vi "LinxI2cRead.vi"(5 "EOF":u8, 6 "Timeout (1000 ms)":u16=1000, 7 "I2C Channel":u8, 8 "Error In":errorcluster, 9 "Num Bytes":u8, 10 "Slave Address":u8, 11 "LINX Resource":T1) -> (0 "Error Out":errorcluster, 2 "Data":u8[](array[numeric]), 3 "LINX Resource":T1)   [LabVIEW 2019, in "LMH-LINX.lvlib" / "Local IO.lvlib"]
uses:
  <vilib>/MakerHub/LINX/Private/Local IO/Local IO.lvlib
  <vilib>/MakerHub/LINX/Private/Type Defs/LINX Ref.ctl
  <vilib>/MakerHub/LINX/Private/Type Defs/Platform.ctl
  <vilib>/MakerHub/LINX/Private/Type Defs/Interface.ctl
  <vilib>/MakerHub/LINX/Private/Device/Type Defs/LINX Device Config.ctl
  <vilib>/MakerHub/LINX/Private/Device/Type Defs/TCP Config.ctl
  <vilib>/MakerHub/LINX/Private/Device/Type Defs/Channels.ctl
  <vilib>/MakerHub/LINX/LMH-LINX.lvlib
  <vilib>/MakerHub/LINX/Private/Type Defs/Channel FGV States.ctl
  <vilib>/myRIO/Instrument Drivers/Onboard IO/I2C/typedefs/I2C Transfer Rate.ctl
  <vilib>/myRIO/Instrument Drivers/Onboard IO/I2C/typedefs/I2C Configuration.ctl
  <vilib>/myRIO/Common/Instrument Driver Framework/myRIO v1.0/I2C/typedefs/I2C Channels Enum.ctl
  <vilib>/myRIO/Common/Instrument Driver Framework/Utilities/typedefs/Generic FPGA Reference.ctl
  <vilib>/myRIO/Common/Instrument Driver Framework/Utilities/typedefs/myRIO v1.0 Reference.ctl
  <vilib>/myRIO/Common/Instrument Driver Framework/Utilities/typedefs/Hardware Version Enum.ctl
  <vilib>/myRIO/Common/Instrument Driver Framework/Utilities/typedefs/myRIO Generic Hardware Reference.ctl
  <vilib>/myRIO/Instrument Drivers/Onboard IO/I2C/typedefs/I2C Reference.ctl
  <vilib>/MakerHub/LINX/Resources/liblinxdevice.dll
  <vilib>/MakerHub/LINX/Private/Device/Device.lvlib
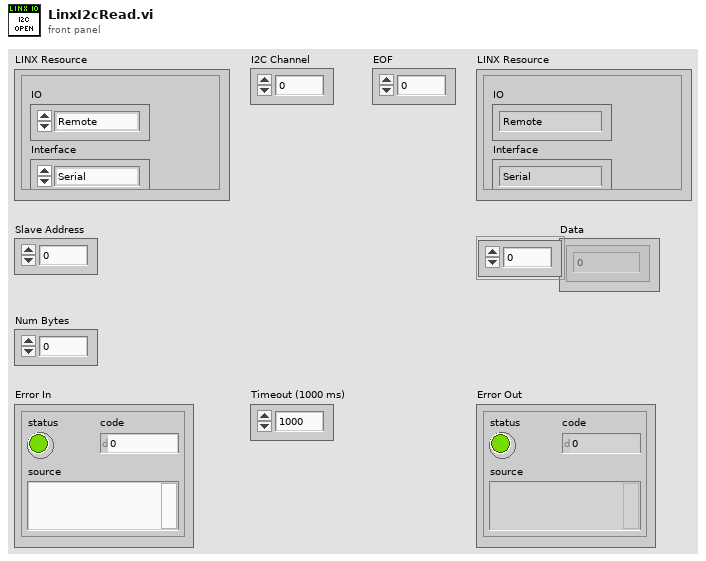
[diagram p1: front panel]
types:
  T1 = typedef "LMH-LINX.lvlib/LINX Ref.ctl" = cluster{"IO":T2, "Interface":T3, "LINX Device Config":T4}
  T2 = typedef "LMH-LINX.lvlib/Platform.ctl" = enum16{"Remote", "Local"}
  T3 = typedef "LMH-LINX.lvlib/Interface.ctl" = enum16{"Serial", "TCP"}
  T4 = typedef "LMH-LINX.lvlib/Device.lvlib/LINX Device Config.ctl" = cluster{"Interface":T3, "COM Port":refnum<visa-resource-name>, "TCP Configuration":T5, "Device Family":u8, "Device ID":u8, "Device Name":string, "TCP Ref":refnum<k5>, "Channels":T6}
  T5 = typedef "LMH-LINX.lvlib/Device.lvlib/TCP Config.ctl" = cluster{"IP Address":string, "Port":u16}
  T6 = typedef "LMH-LINX.lvlib/Channels.ctl" = cluster{"DI":u8[], "DO":u8[], "AI":u8[], "AO":u8[], "PWM":u8[], "QE":u8[], "UART":u8[], "I2C 2":u8[], "SPI":u8[], "CAN":u8[], "Servo":u8[], "AI Ref (V)":dbl, "AI Resolution (Bits)":u8, "AO Ref (V)":dbl, "AO Resolution (Bits)":u8}
  T7 = typedef "I2C.lvlib/I2C Reference.ctl" = cluster{"myRIO Reference":T8, "I2C Channels Enum":T12, "I2C Configuration":T13}
  T8 = typedef "myRIO Generic Hardware Reference.ctl" = cluster{"myRIO Model":T9, "myRIO Hardware Reference":T10}
  T9 = typedef "Hardware Version Enum.ctl" = enum16{"Unknown", "myRIO-1900", "myRIO-1950"}
  T10 = typedef "myRIO v1.0 Reference.ctl" = cluster{"Generic FPGA Reference":T11, "Allow multiple opens":bool}
  T11 = typedef "Generic FPGA Reference.ctl" = refnum<k20>
  T12 = typedef "I2C Channels Enum.ctl" = enum16{"Not Connected", "A/I2C", "B/I2C"}
  T13 = typedef "I2C.lvlib/I2C Configuration.ctl" = cluster{"I2C Transfer Rate":T14}
  T14 = typedef "I2C.lvlib/I2C Transfer Rate.ctl" = enum16{"Standard mode (100 kbps)", "Fast mode (400 kbps)"}
  T15 = typedef "LMH-LINX.lvlib/Channel FGV States.ctl" = enum16{"Initialize", "Get", "Set"}
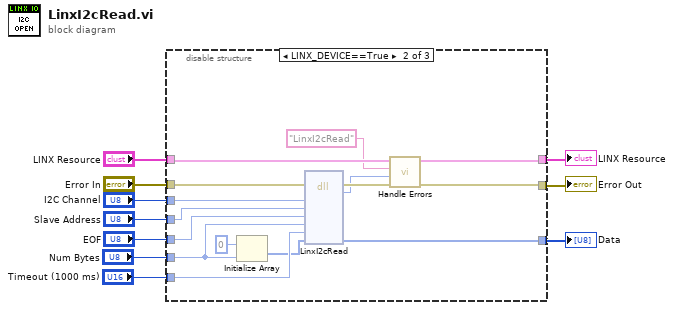
[diagram p0: block diagram]
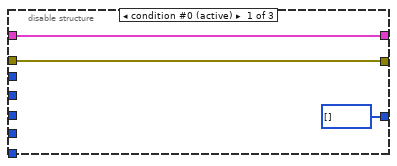
[diagram p2: hidden frame]
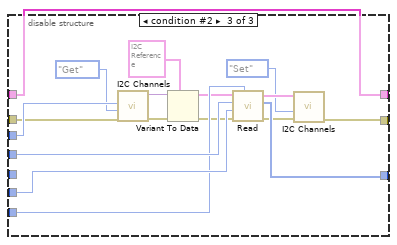
[diagram p3: hidden frame]
diagram:
  n1 = disable-structure shown="LINX_DEVICE==True" {
    disable-tunnel: "LINX Resource" -> [w13 w27 w44]
    disable-tunnel: "Error In" -> [w12 w28 w42]
    disable-tunnel: [w12 w25 w45] -> w8
    disable-tunnel: [w13 w26 w44] -> w7
    disable-tunnel: "I2C Channel" -> [_ w21 w43]
    disable-tunnel: "Slave Address" -> [_ w20 w41]
    disable-tunnel: "EOF" -> [_ w19 _]
    disable-tunnel: "Timeout (1000 ms)" -> [_ w18 w39]
    disable-tunnel: "Num Bytes" -> [_ w15 w40]
    disable-tunnel: [u8[] [] ("Data") w14 w38] -> w1
    frame condition #0 (active) {
    }
    frame condition #1 {
      n2 = Initialize Array(u8 0 ("dimension size"), w15) -> (w16:u8[])
      n3 = dll-call lib="E:/lv2019/dist/vi.lib/MakerHub/LINX/Resources/liblinxdevice.*" fn="LinxI2cRead"(error in=w28, "channel"=w21, "slaveAddress"=w20, "eofConfig"=w19, "numBytes"=w15, "timeout"=w18, "recBuffer"=w16) -> (error out=w24:errorcluster, "LinxStatus"=w23:i32, "recBuffer"=w14:u8[])  [unwired: 7 in, 1 out]
      n4 = call <vilib>:"Handle Errors.vi"("Error In"=w24, "LinxStatus"=w23, "Function Name"="LinxI2cRead", "LINX Resource"=w27) -> ("Error Out"=w25:errorcluster, "LINX Resource"=w26:T1)  [unwired: 6 in]
    }
    frame condition #2 {
      n5 = call <vilib>:"I2C Channels.vi"("Error In"=w42, "Channel State"=Channel_FGV_States."Get", "Channel Number"=w43) -> ("Error Out"=w31:errorcluster, "I2C Channel"=w32:variant)  [unwired: 7 in]
      n6 = Variant To Data(error in=w31, type=T7 {"myRIO Reference"={"myRIO Model"=enum."Unknown", "myRIO Hardware Reference"={"Generic FPGA Reference"=refnum, "Allow multiple opens"=FALSE}}, "I2C Channels Enum"=enum."Not Connected", "I2C Configuration"={"I2C Transfer Rate"=enum."Standard mode (100 kbps)"}}, Variant=w32) -> (data=w37:T7, error out=w36:errorcluster)
      n7 = call <vilib>:"Read.vi"("Timeout ms (1000)"=w39, "error in (no error)"=w36, "Byte Count"=w40, "Slave Address (7-bit)"=w41, "I2C Ref In"=w37) -> ("error out"=w34:errorcluster, "Bytes Read"=w38:u8[], "I2C Ref Out"=w33:T7)  [unwired: 3 in]
      n8 = call <vilib>:"I2C Channels.vi"("Error In"=w34, "Channel State"=Channel_FGV_States."Set", "I2C Channel"=w33) -> ("Error Out"=w45:errorcluster)  [unwired: 7 in, 1 out]
    }
  }
  "Error Out" <- w8
  "LINX Resource" <- w7
  "Data" <- w1
